vi "Control Structure.vi"(8 "error in (no error)":errorcluster, 11 "Vessel in":refnum<class "Vessel.lvclass">) -> (0 "error out":errorcluster, 3 "Vessel out":refnum<class "Vessel.lvclass">)   [LabVIEW 2014, in "Vessel.lvclass"]
doc: "This is the main running method that runs the control loop."
uses:
  Vessel.lvclass
  Supervisor/Supervisor.lvclass
  Observer/Observer.lvclass
  Guidance/Guidance.lvclass
  Controller/Controller.lvclass
  Thrust Allocation/Thrust Allocation.lvclass
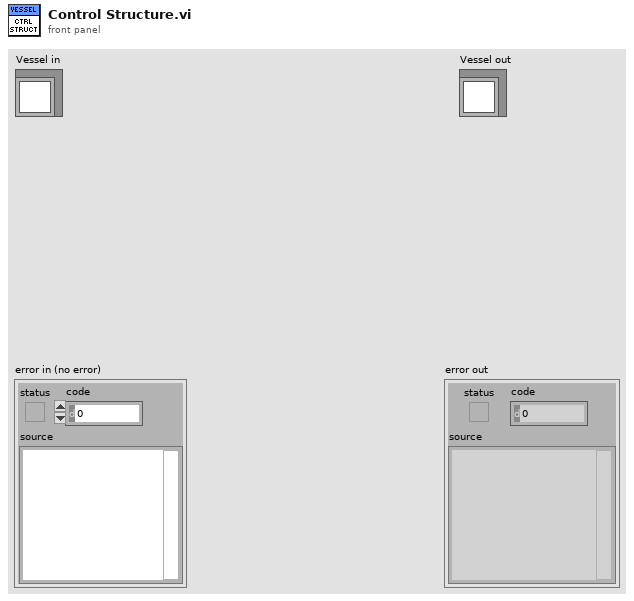
[diagram p1: front panel]
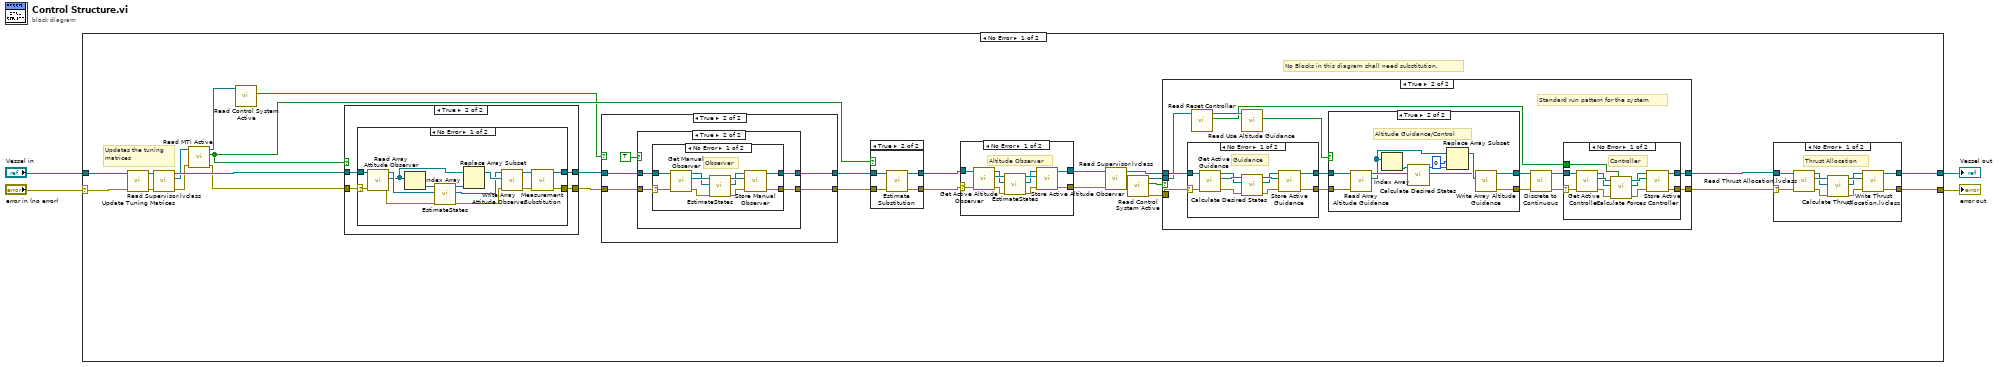
[diagram p0: block diagram]
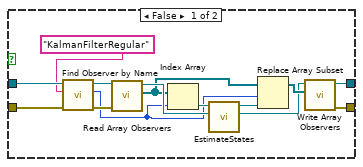
[diagram p2: hidden frame]
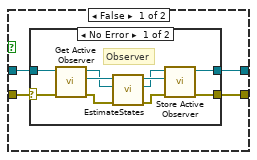
[diagram p3: hidden frame]
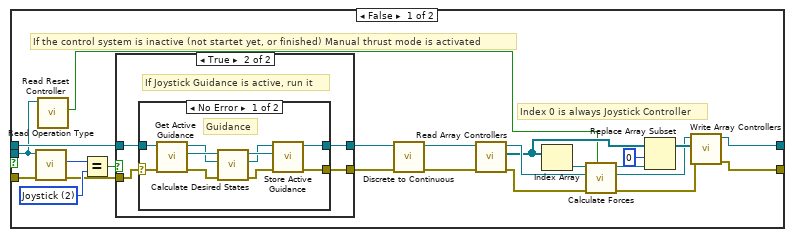
[diagram p9: hidden frame]
diagram:
  n1 = case shown="No Error" "error in (no error)" {
    selector: "error in (no error)" -> [w26 w231]
    tunnel: [w13 w231] -> w3
    tunnel: [w14 w230] -> w1
    tunnel: "Vessel in" -> [w27 w230]
    frame No Error {
      # "Updates the tuning\nmatrices"
      # "No Blocks in this diagram shall need substitution."
      n2 = call-dynamic "Update Tuning Matrices.vi"("error in (no error)"=w26, "Vessel in"=w27) -> ("error out"=w22:errorcluster, "Vessel out"=w24:refnum<class "Vessel.lvclass">)  [unwired: 8 in]
      n3 = call "Read Supervisor.lvclass.vi"("error in (no error)"=w22, "Vessel in"=w24) -> ("error out"=w19:errorcluster, "Supervisor.lvclass"=w21:refnum<class "Supervisor.lvclass">, "Vessel out"=w23:refnum<class "Vessel.lvclass">)  [unwired: 7 in]
      n4 = call-dynamic "Read MTi Active.vi"("error in (no error)"=w19, "Supervisor in"=w21) -> ("error out"=w18:errorcluster, "MTi Active"=w20:bool, "Supervisor out"=w17:refnum<class "Supervisor.lvclass">)  [unwired: 7 in]
      n5 = call-dynamic "Read Control System Active.vi"("Supervisor in"=w17) -> ("Control System Active"=w16:bool)  [unwired: 8 in, 2 out]
      n6 = case shown="True" w20 {
        tunnel: [w92 w96] -> w15
        tunnel: [w91 w95] -> w25
        tunnel: w23 -> [w92 w94]
        tunnel: w18 -> [w91 w93]
        frame False {
        }
        frame True {
          n7 = case shown="No Error" w93 {
            selector: w93 -> [w109 w111]
            tunnel: w94 -> [w110 w112]
            tunnel: [w101 w112] -> w96
            tunnel: [w97 w111] -> w95
            frame No Error {
              n8 = call-dynamic "Read Array Attitude Observer.vi"("error in (no error)"=w109, "Vessel in"=w110) -> ("error out"=w100:errorcluster, "Array Attitude Observer"=w105:refnum<class "Observer.lvclass">[], "Vessel out"=w107:refnum<class "Vessel.lvclass">)  [unwired: 7 in]
              n9 = Index Array(array=w105) -> (element=w108:refnum<class "Observer.lvclass">)  [unwired: 1 in]
              n10 = call-dynamic "EstimateStates.vi"("error in (no error)"=w100, "Vessel In"=w107, "Observer in"=w108) -> ("error out"=w99:errorcluster, "Vessel Out"=w103:refnum<class "Vessel.lvclass">, "Observer out"=w106:refnum<class "Observer.lvclass">)  [unwired: 6 in]
              n11 = Replace Array Subset(array=w105, new element=w106) -> (w104:refnum<class "Observer.lvclass">[])  [unwired: 1 in]
              n12 = call-dynamic "Write Array Attitude Observer.vi"("error in (no error)"=w99, "Array Attitude Observer"=w104, "Vessel in"=w103) -> ("error out"=w98:errorcluster, "Vessel out"=w102:refnum<class "Vessel.lvclass">)  [unwired: 7 in]
              n13 = call-dynamic "Measurement Substitution.vi"("error in (no error)"=w98, "Vessel in"=w102) -> ("error out"=w97:errorcluster, "Vessel out"=w101:refnum<class "Vessel.lvclass">)  [unwired: 8 in]
            }
            frame Error {
            }
          }
        }
      }
      n14 = case shown="True" w16 {
        tunnel: [w35 w52] -> w10
        tunnel: [w36 w51] -> w11
        tunnel: w15 -> [w47 w50]
        tunnel: w25 -> [w46 w49]
        frame False {
          n15 = call-dynamic "Find Observer by Name.vi"("error in (no error)"=w46, "Observer Name"="KalmanFilterRegular", "Vessel in"=w47) -> ("error out"=w43:errorcluster, "Index"=w34:i32, "Vessel out"=w44:refnum<class "Vessel.lvclass">)  [unwired: 6 in]
          n16 = call-dynamic "Read Array Observers.vi"("error in (no error)"=w43, "Vessel in"=w44) -> ("Array Observers"=w39:refnum<class "Observer.lvclass">[], "Vessel out"=w41:refnum<class "Vessel.lvclass">)  [unwired: 7 in, 1 out]
          n17 = Index Array(array=w39, index=w34) -> (element=w42:refnum<class "Observer.lvclass">)
          n18 = call-dynamic "EstimateStates.vi"("Vessel In"=w41, "Observer in"=w42) -> ("Vessel Out"=w37:refnum<class "Vessel.lvclass">, "Observer out"=w40:refnum<class "Observer.lvclass">)  [unwired: 7 in, 1 out]
          n19 = Replace Array Subset(array=w39, new element=w40, index=w34) -> (w38:refnum<class "Observer.lvclass">[])
          n20 = call-dynamic "Write Array Observers.vi"("Array Observers"=w38, "Vessel in"=w37) -> ("error out"=w35:errorcluster, "Vessel out"=w36:refnum<class "Vessel.lvclass">)  [unwired: 8 in]
        }
        frame True {
          n21 = case shown="True" TRUE {
            tunnel: [w56 w70] -> w52
            tunnel: [w55 w69] -> w51
            tunnel: w50 -> [w54 w72]
            tunnel: w49 -> [w53 w71]
            frame False {
              n22 = case shown="No Error" w53 {
                selector: w53 -> [w60 w68]
                tunnel: [w62 w67] -> w55
                tunnel: w54 -> [w61 w67]
                tunnel: [w57 w68] -> w56
                frame No Error {
                  # "Observer"
                  n23 = call-dynamic "Get Active Observer.vi"("error in (no error)"=w60, "Vessel in"=w61) -> ("error out"=w59:errorcluster, "Active Observer"=w66:refnum<class "Observer.lvclass">, "Vessel out"=w65:refnum<class "Vessel.lvclass">)  [unwired: 7 in]
                  n24 = call-dynamic "EstimateStates.vi"("error in (no error)"=w59, "Vessel In"=w65, "Observer in"=w66) -> ("error out"=w58:errorcluster, "Vessel Out"=w63:refnum<class "Vessel.lvclass">, "Observer out"=w64:refnum<class "Observer.lvclass">)  [unwired: 6 in]
                  n25 = call-dynamic "Store Active Observer.vi"("error in (no error)"=w58, "Observer In"=w64, "Vessel in"=w63) -> ("error out"=w57:errorcluster, "Vessel out"=w62:refnum<class "Vessel.lvclass">)  [unwired: 7 in]
                }
                frame Error {
                }
              }
            }
            frame True {
              n26 = case shown="No Error" w71 {
                selector: w71 -> [w76 w84]
                tunnel: [w78 w83] -> w69
                tunnel: w72 -> [w77 w83]
                tunnel: [w73 w84] -> w70
                frame No Error {
                  # "Observer"
                  n27 = call-dynamic "Get Manual Observer.vi"("error in (no error)"=w76, "Vessel in"=w77) -> ("error out"=w75:errorcluster, "Active Observer"=w82:refnum<class "Observer.lvclass">, "Vessel out"=w81:refnum<class "Vessel.lvclass">)  [unwired: 7 in]
                  n28 = call-dynamic "EstimateStates.vi"("error in (no error)"=w75, "Vessel In"=w81, "Observer in"=w82) -> ("error out"=w74:errorcluster, "Vessel Out"=w79:refnum<class "Vessel.lvclass">, "Observer out"=w80:refnum<class "Observer.lvclass">)  [unwired: 6 in]
                  n29 = call-dynamic "Store Manual Observer.vi"("error in (no error)"=w74, "Observer In"=w80, "Vessel in"=w79) -> ("error out"=w73:errorcluster, "Vessel out"=w78:refnum<class "Vessel.lvclass">)  [unwired: 7 in]
                }
                frame Error {
                }
              }
            }
          }
        }
      }
      n30 = case shown="True" w20 {
        tunnel: [w86 w90] -> w9
        tunnel: w11 -> [w86 w89]
        tunnel: [w85 w88] -> w8
        tunnel: w10 -> [w85 w87]
        frame False {
        }
        frame True {
          n31 = call-dynamic "Estimate Substitution.vi"("error in (no error)"=w87, "Vessel in"=w89) -> ("error out"=w88:errorcluster, "Vessel out"=w90:refnum<class "Vessel.lvclass">)  [unwired: 8 in]
        }
      }
      n32 = case shown="No Error" w8 {
        selector: w8 -> [w214 w217]
        tunnel: [w212 w217] -> w6
        tunnel: w9 -> [w215 w216]
        tunnel: [w213 w216] -> w7
        frame No Error {
          # "Altitude Observer"
          n33 = call-dynamic "Get Active Altitude Observer.vi"("error in (no error)"=w214, "Vessel in"=w215) -> ("error out"=w211:errorcluster, "Active Altitude Observer"=w209:refnum<class "Observer.lvclass">, "Vessel out"=w207:refnum<class "Vessel.lvclass">)  [unwired: 7 in]
          n34 = call-dynamic "EstimateStates.vi"("error in (no error)"=w211, "Vessel In"=w207, "Observer in"=w209) -> ("error out"=w210:errorcluster, "Vessel Out"=w206:refnum<class "Vessel.lvclass">, "Observer out"=w208:refnum<class "Observer.lvclass">)  [unwired: 6 in]
          n35 = call-dynamic "Store Active Altitude Observer.vi"("error in (no error)"=w210, "Altitude Observer In"=w208, "Vessel in"=w206) -> ("error out"=w212:errorcluster, "Vessel out"=w213:refnum<class "Vessel.lvclass">)  [unwired: 7 in]
        }
        frame Error {
        }
      }
      n36 = call "Read Supervisor.lvclass.vi"("error in (no error)"=w6, "Vessel in"=w7) -> ("error out"=w31:errorcluster, "Supervisor.lvclass"=w32:refnum<class "Supervisor.lvclass">, "Vessel out"=w33:refnum<class "Vessel.lvclass">)  [unwired: 7 in]
      n37 = call-dynamic "Read Control System Active.vi"("error in (no error)"=w31, "Supervisor in"=w32) -> ("error out"=w30:errorcluster, "Control System Active"=w29:bool, "Supervisor out"=w28:refnum<class "Supervisor.lvclass">)  [unwired: 7 in]
      n38 = case shown="True" w29 {
        tunnel: [w120 w167] -> w12
        tunnel: [w119 w166] -> w5
        tunnel: w33 -> [w131 w165]
        tunnel: w30 -> [w135 w164]
        tunnel: w28 -> [w118 w159]
        frame False {
          w133 = u16 2 items=["Tracking", "DP", "Joystick"] ("Operation Type")
          # "If the control system is inactive (not startet yet, or finished) Manual thrust mode is activated"
          # "Index 0 is always Joystick Controller"
          n39 = call-dynamic "Read Operation Type.vi"("error in (no error)"=w135, "Supervisor in"=w118) -> ("error out"=w130:errorcluster, "Operation Type"=w134:u16)  [unwired: 7 in, 1 out]
          n40 = call-dynamic "Read Reset Controller.vi"("Supervisor in"=w118) -> ("Reset Controller"=w117:bool)  [unwired: 8 in, 2 out]
          n41 = Equal?(x=w134, y=w133) -> (x = y?=w132:bool)
          n42 = case shown="True" w132 {
            tunnel: w131 -> [w137 w141]
            tunnel: w130 -> [w136 w140]
            tunnel: [w137 w139] -> w116
            tunnel: [w136 w138] -> w113
            frame False {
            }
            frame True {
              # "If Joystick Guidance is active, run it"
              n43 = case shown="No Error" w140 {
                selector: w140 -> [w148 w153]
                tunnel: w141 -> [w151 w152]
                tunnel: [w146 w152] -> w139
                tunnel: [w145 w153] -> w138
                frame No Error {
                  # "Guidance"
                  n44 = call-dynamic "Get Active Guidance.vi"("error in (no error)"=w148, "Vessel in"=w151) -> ("error out"=w147:errorcluster, "Guidance Out"=w150:refnum<class "Guidance.lvclass">, "Vessel out"=w149:refnum<class "Vessel.lvclass">)  [unwired: 7 in]
                  n45 = call-dynamic "Calculate Desired States.vi"("error in (no error)"=w147, "Vessel In"=w149, "CJ Guidance in"=w150) -> ("error out"=w142:errorcluster, "Vessel Out"=w143:refnum<class "Vessel.lvclass">, "CJ Guidance out"=w144:refnum<class "Guidance.lvclass">)  [unwired: 6 in]
                  n46 = call-dynamic "Store Active Guidance.vi"("error in (no error)"=w142, "Guidance In"=w144, "Vessel in"=w143) -> ("error out"=w145:errorcluster, "Vessel out"=w146:refnum<class "Vessel.lvclass">)  [unwired: 7 in]
                }
                frame Error {
                }
              }
            }
          }
          n47 = call-dynamic "Discrete to Continuous.vi"("error in (no error)"=w113, "Vessel in"=w116) -> ("error out"=w114:errorcluster, "Vessel out"=w115:refnum<class "Vessel.lvclass">)  [unwired: 8 in]
          n48 = call "Read Array Controllers.vi"("error in (no error)"=w114, "Vessel in"=w115) -> ("error out"=w127:errorcluster, "Array Controllers"=w125:refnum<class "Controller.lvclass">[], "Vessel out"=w128:refnum<class "Vessel.lvclass">)  [unwired: 7 in]
          n49 = Index Array(array=w125) -> (element=w129:refnum<class "Controller.lvclass">)  [unwired: 1 in]
          n50 = call-dynamic "Calculate Forces.vi"("Integrator Reset"=w117, "error in (no error)"=w127, "Vessel in"=w128, "Controller in"=w129) -> ("error out"=w121:errorcluster, "Vessel out"=w122:refnum<class "Vessel.lvclass">, "Controller out"=w126:refnum<class "Controller.lvclass">)  [unwired: 5 in]
          n51 = Replace Array Subset(array=w125, new element=w126, index=0) -> (w123:refnum<class "Controller.lvclass">[])
          n52 = call "Write Array Controllers.vi"("error in (no error)"=w121, "Array Controllers"=w123, "Vessel in"=w122) -> ("error out"=w119:errorcluster, "Vessel out"=w120:refnum<class "Vessel.lvclass">)  [unwired: 7 in]
        }
        frame True {
          # "Standard run pattern for the system"
          n53 = case shown="No Error" w164 {
            selector: w164 -> [w200 w205]
            tunnel: w165 -> [w203 w204]
            tunnel: [w198 w204] -> w163
            tunnel: [w197 w205] -> w162
            frame No Error {
              # "Guidance"
              n54 = call-dynamic "Get Active Guidance.vi"("error in (no error)"=w200, "Vessel in"=w203) -> ("error out"=w199:errorcluster, "Guidance Out"=w202:refnum<class "Guidance.lvclass">, "Vessel out"=w201:refnum<class "Vessel.lvclass">)  [unwired: 7 in]
              n55 = call-dynamic "Calculate Desired States.vi"("error in (no error)"=w199, "Vessel In"=w201, "CJ Guidance in"=w202) -> ("error out"=w194:errorcluster, "Vessel Out"=w195:refnum<class "Vessel.lvclass">, "CJ Guidance out"=w196:refnum<class "Guidance.lvclass">)  [unwired: 6 in]
              n56 = call-dynamic "Store Active Guidance.vi"("error in (no error)"=w194, "Guidance In"=w196, "Vessel in"=w195) -> ("error out"=w197:errorcluster, "Vessel out"=w198:refnum<class "Vessel.lvclass">)  [unwired: 7 in]
            }
            frame Error {
            }
          }
          n57 = call-dynamic "Read Reset Controller.vi"("Supervisor in"=w159) -> ("Reset Controller"=w158:bool, "Supervisor out"=w160:refnum<class "Supervisor.lvclass">)  [unwired: 8 in, 1 out]
          n58 = call-dynamic "Read Use Altitude Guidance.vi"("Supervisor in"=w160) -> ("Use Altitude Guidance"=w161:bool)  [unwired: 8 in, 2 out]
          n59 = case shown="True" w161 {
            tunnel: w163 -> [w169 w173]
            tunnel: [w169 w172] -> w155
            tunnel: [w168 w171] -> w156
            tunnel: w162 -> [w168 w170]
            frame False {
            }
            frame True {
              # "Altitude Guidance/Control"
              n60 = call-dynamic "Read Array Altitude Guidance.vi"("error in (no error)"=w170, "Vessel in"=w173) -> ("Array Altitude Guidance"=w177:refnum<class "Guidance.lvclass">[], "Vessel out"=w179:refnum<class "Vessel.lvclass">)  [unwired: 7 in, 1 out]
              n61 = Index Array(array=w177) -> (element=w180:refnum<class "Guidance.lvclass">)  [unwired: 1 in]
              n62 = call-dynamic "Calculate Desired States.vi"("Vessel In"=w179, "CJ Guidance in"=w180) -> ("Vessel Out"=w174:refnum<class "Vessel.lvclass">, "CJ Guidance out"=w178:refnum<class "Guidance.lvclass">)  [unwired: 7 in, 1 out]
              n63 = Replace Array Subset(array=w177, new element=w178, index=0) -> (w175:refnum<class "Guidance.lvclass">[])
              n64 = call-dynamic "Write Array Altitude Guidance.vi"("Array Altitude Guidance"=w175, "Vessel in"=w174) -> ("error out"=w171:errorcluster, "Vessel out"=w172:refnum<class "Vessel.lvclass">)  [unwired: 8 in]
            }
          }
          n65 = call-dynamic "Discrete to Continuous.vi"("error in (no error)"=w156, "Vessel in"=w155) -> ("error out"=w157:errorcluster, "Vessel out"=w154:refnum<class "Vessel.lvclass">)  [unwired: 8 in]
          n66 = case shown="No Error" w157 {
            selector: w157 -> [w185 w192]
            tunnel: [w187 w193] -> w167
            tunnel: w154 -> [w186 w193]
            tunnel: [w182 w192] -> w166
            tunnel: w158 -> [w181 _]
            frame No Error {
              # "Controller"
              n67 = call-dynamic "Get Active Controller.vi"("error in (no error)"=w185, "Vessel in"=w186) -> ("error out"=w184:errorcluster, "Controller Out"=w191:refnum<class "Controller.lvclass">, "Vessel out"=w189:refnum<class "Vessel.lvclass">)  [unwired: 7 in]
              n68 = call-dynamic "Calculate Forces.vi"("Integrator Reset"=w181, "error in (no error)"=w184, "Vessel in"=w189, "Controller in"=w191) -> ("error out"=w183:errorcluster, "Vessel out"=w188:refnum<class "Vessel.lvclass">, "Controller out"=w190:refnum<class "Controller.lvclass">)  [unwired: 5 in]
              n69 = call-dynamic "Store Active Controller.vi"("error in (no error)"=w183, "Controller In"=w190, "Vessel in"=w188) -> ("error out"=w182:errorcluster, "Vessel out"=w187:refnum<class "Vessel.lvclass">)  [unwired: 7 in]
            }
            frame Error {
            }
          }
        }
      }
      n70 = case shown="No Error" w5 {
        selector: w5 -> [w221 w229]
        tunnel: w12 -> [w227 w228]
        tunnel: [w222 w228] -> w14
        tunnel: [w218 w229] -> w13
        frame No Error {
          # "Thrust Allocation"
          n71 = call "Read Thrust Allocation.lvclass.vi"("error in (no error)"=w221, "Vessel in"=w227) -> ("error out"=w220:errorcluster, "Thrust Allocation.lvclass"=w226:refnum<class "Thrust Allocation.lvclass">, "Vessel out"=w225:refnum<class "Vessel.lvclass">)  [unwired: 7 in]
          n72 = call-dynamic "Calculate Thrust.vi"("error in (no error)"=w220, "Vessel in"=w225, "Thrust Allocation in"=w226) -> ("error out"=w219:errorcluster, "Vessel out"=w223:refnum<class "Vessel.lvclass">, "Thrust Allocation out"=w224:refnum<class "Thrust Allocation.lvclass">)  [unwired: 6 in]
          n73 = call "Write Thrust Allocation.lvclass.vi"("error in (no error)"=w219, "Thrust Allocation.lvclass"=w224, "Vessel in"=w223) -> ("error out"=w218:errorcluster, "Vessel out"=w222:refnum<class "Vessel.lvclass">)  [unwired: 7 in]
        }
        frame Error {
        }
      }
    }
    frame Error {
    }
  }
  "error out" <- w3
  "Vessel out" <- w1
